vi "Memory.Pointer.Numeric.Size to Count.vi"(8 "error in (no error)":errorcluster, 10 "size":u64 format="%d bytes", 11 "Numeric Pointer in":refnum<class "Memory.Pointer.Numeric.lvclass">) -> (0 "error out":errorcluster, 2 "count":u64, 3 "Numeric Pointer out":refnum<class "Memory.Pointer.Numeric.lvclass">)   [LabVIEW 2016, in "LabVIEW Memory Manager.lvlib" / "Memory.Pointer.Numeric.lvclass"]
uses:
  Memory.Pointer.Numeric.lvclass
  Memory.Pointer.Numeric.lvclass/Memory.Pointer.Numeric.ctl
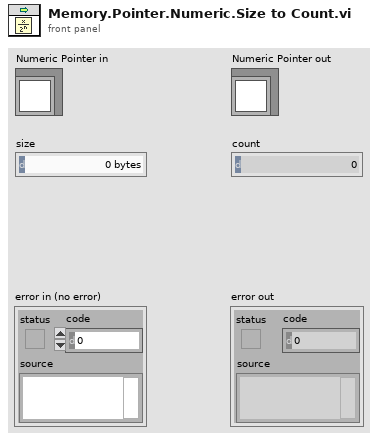
[diagram p1: front panel]
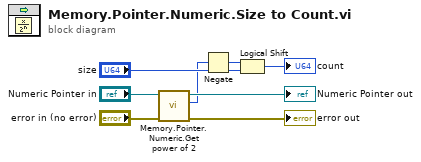
[diagram p0: block diagram]
diagram:
  n1 = call "Memory.Pointer.Numeric.Get power of 2.vi"("error in (no error)"="error in (no error)", "Memory.Pointer.Numeric in"="Numeric Pointer in") -> ("error out"=→"error out":errorcluster, "power of 2"=w1:i16, "Memory.Pointer.Numeric out"=→"Numeric Pointer out":refnum<class "Memory.Pointer.Numeric.lvclass">)  [unwired: 7 in]
  n2 = Negate(x=w1) -> (-x=w2:i16)
  n3 = Logical Shift(y=w2, x="size") -> (x << y=→"count":u64)
